vi "Kolmogan main.vi"(8 "Error In":errorcluster, 11 "Name":string) -> (0 "Error Out":errorcluster)   [LabVIEW 2019, in "Kolmogan Library 1.lvlib"]
uses:
  Kolmogan Library 1.lvlib
  <vilib>/NI/Modbus Library/API/Wrapper/Create TCP Master.vi
  <vilib>/regexp/Match Regular Expression.xnode
  <vilib>/NI/Modbus Library/API/Master/Modbus Master.lvclass
  Queue/Queue.lvlib
  Data Error Notifier/Data and Error Notifier.lvlib
  <vilib>/NI/Modbus Library/API/Wrapper/API Main.lvlib
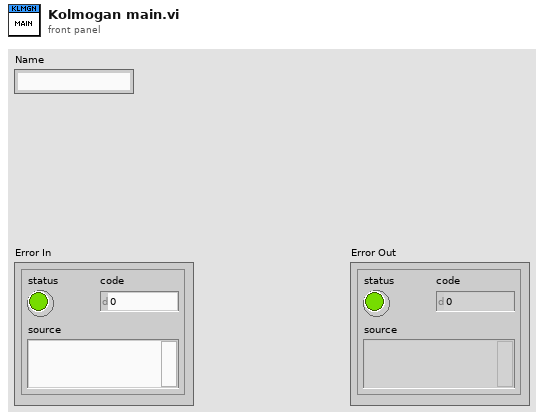
[diagram p1: front panel]
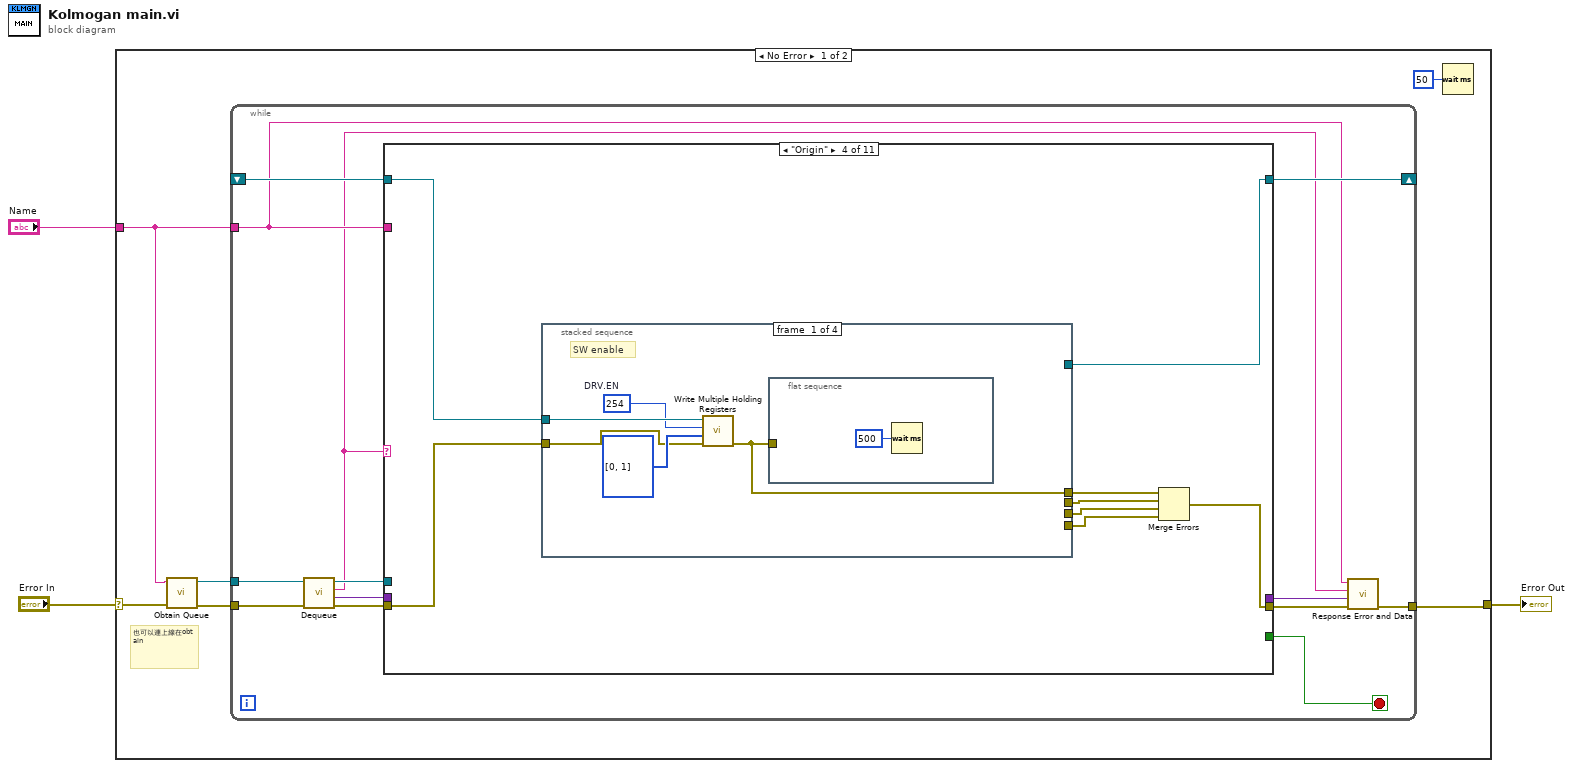
[diagram p0: block diagram]
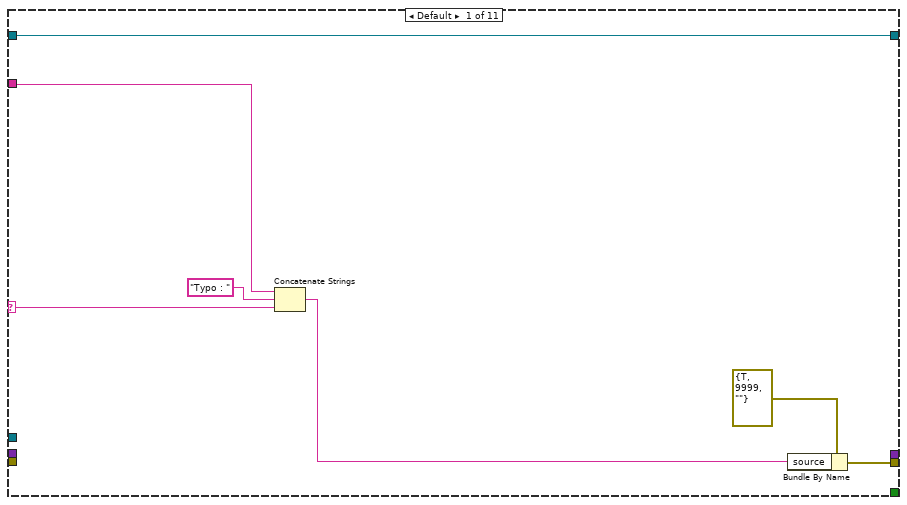
[diagram p2: hidden frame]
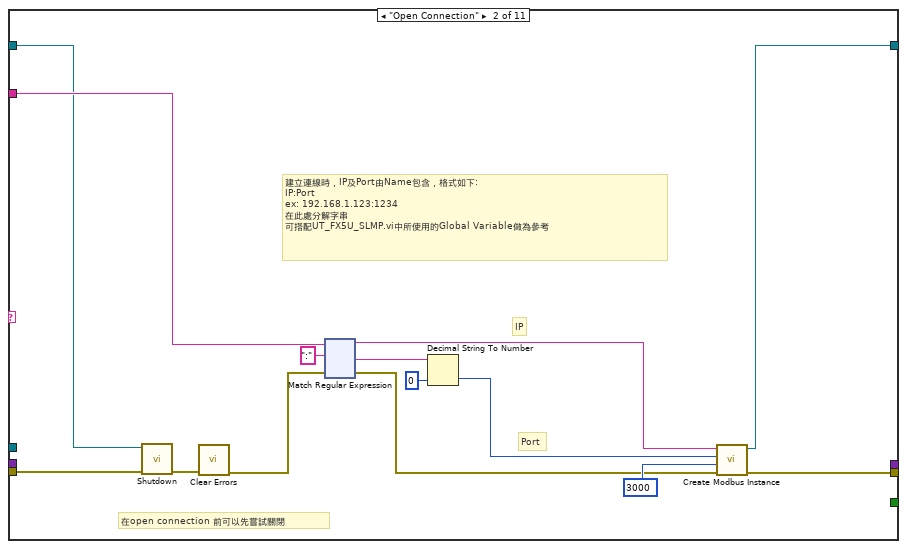
[diagram p3: hidden frame]
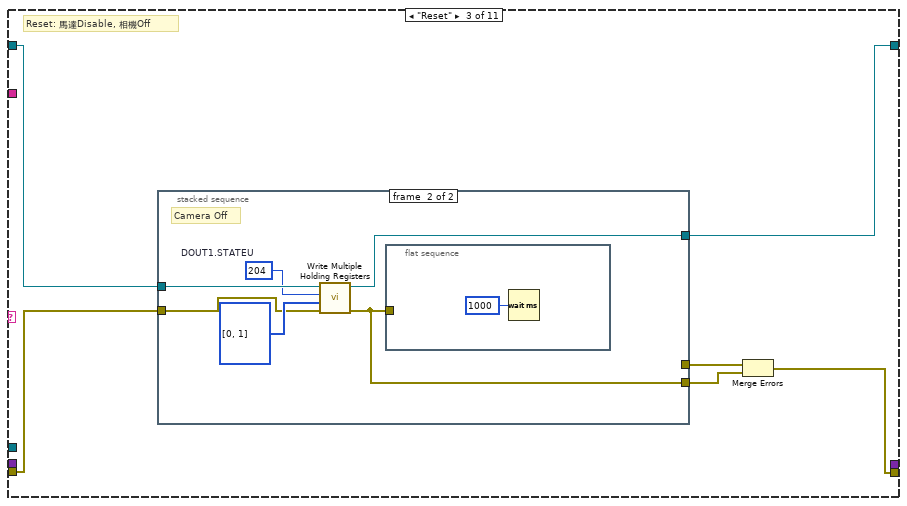
[diagram p4: hidden frame]
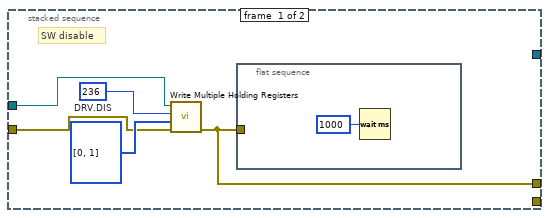
[diagram p5: hidden frame]
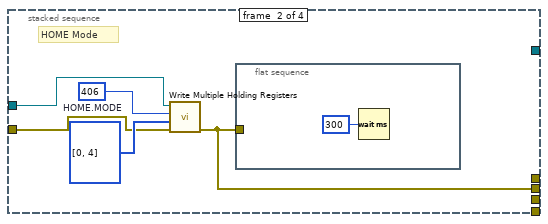
[diagram p6: hidden frame]
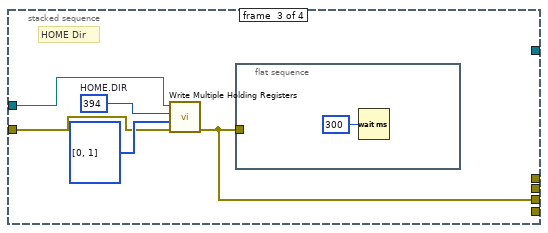
[diagram p7: hidden frame]
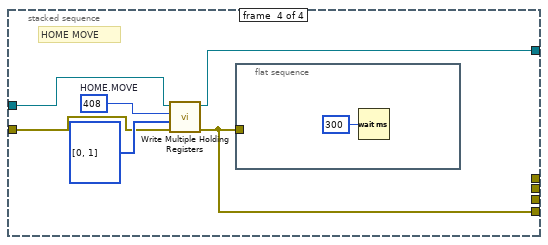
[diagram p8: hidden frame]
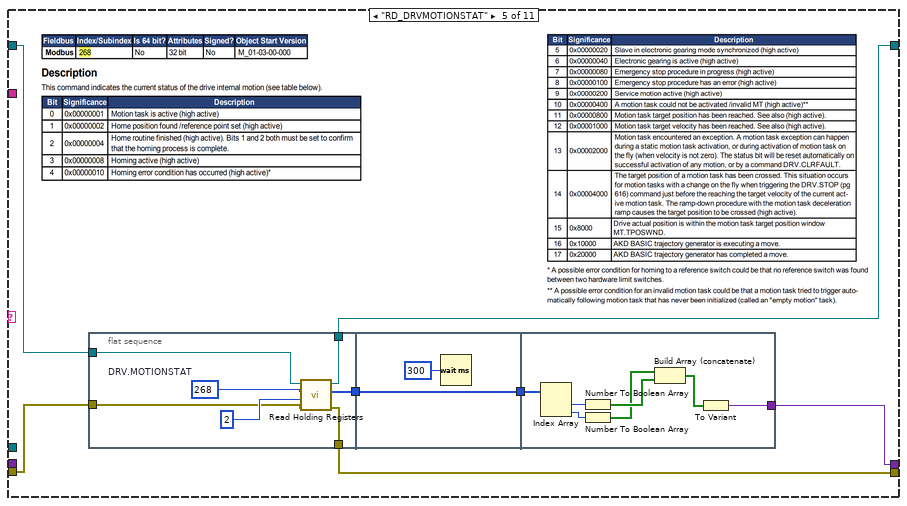
[diagram p9: hidden frame]
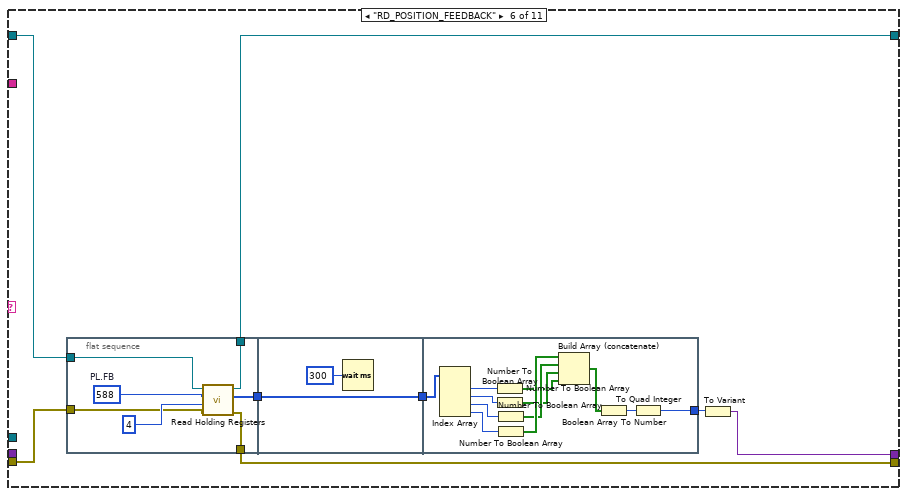
[diagram p10: hidden frame]
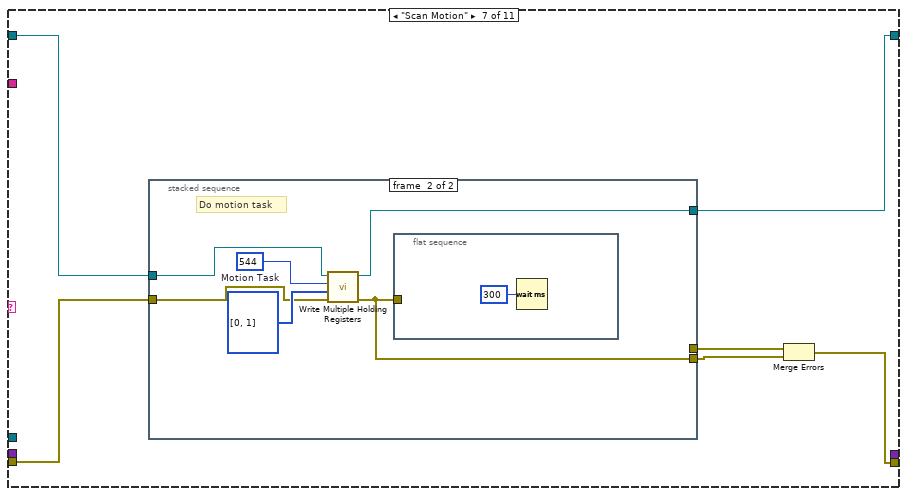
[diagram p11: hidden frame]
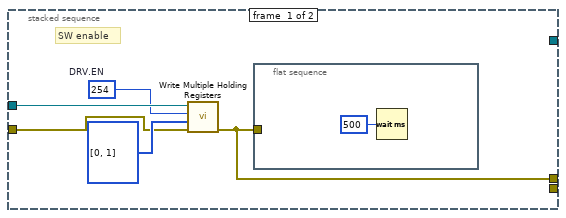
[diagram p12: hidden frame]
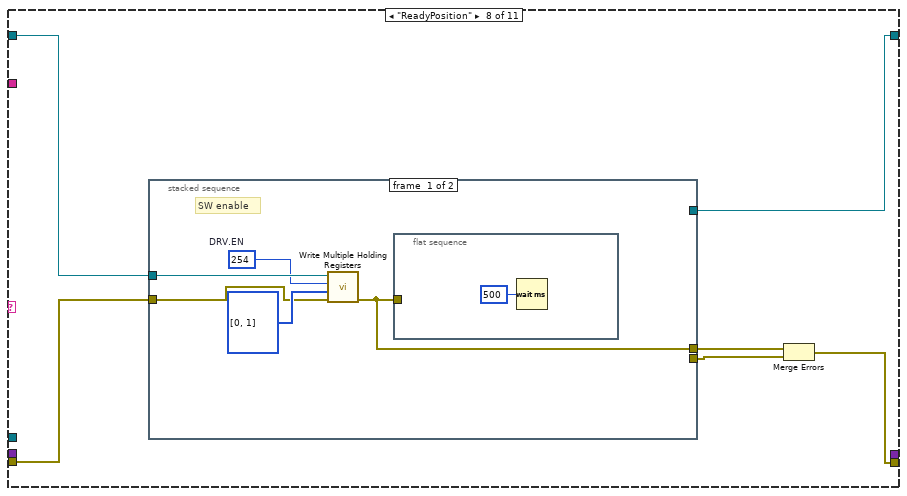
[diagram p13: hidden frame]
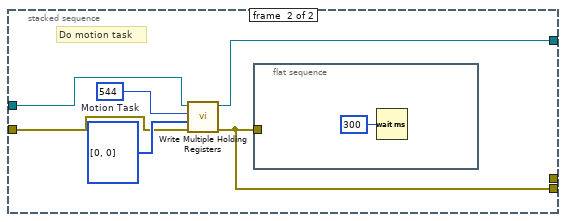
[diagram p14: hidden frame]
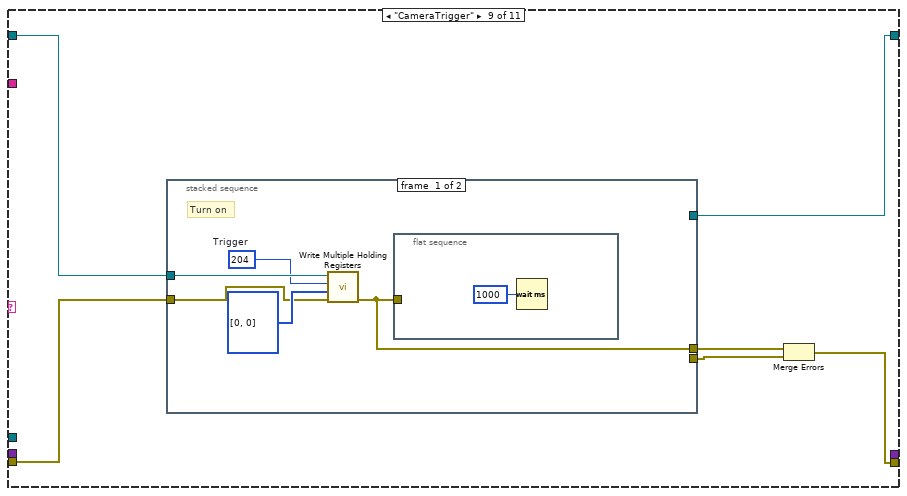
[diagram p15: hidden frame]
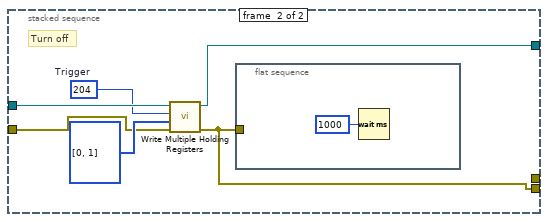
[diagram p16: hidden frame]
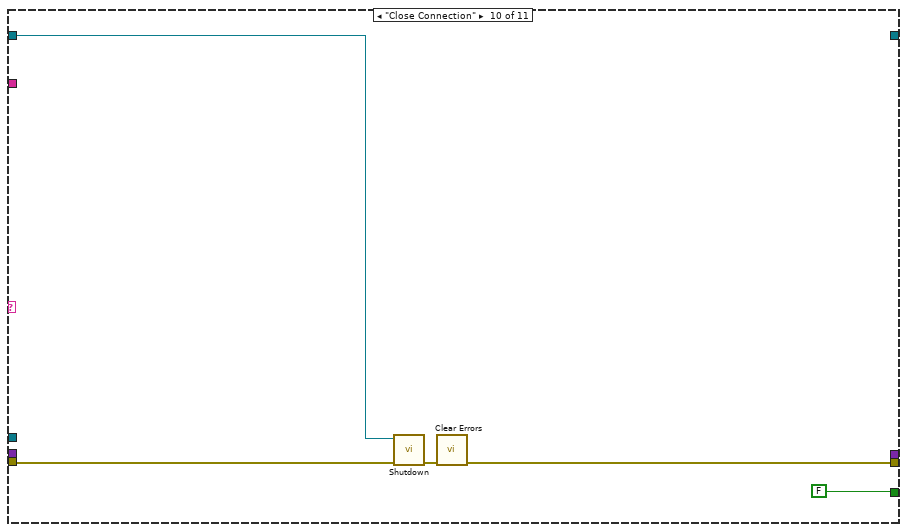
[diagram p17: hidden frame]
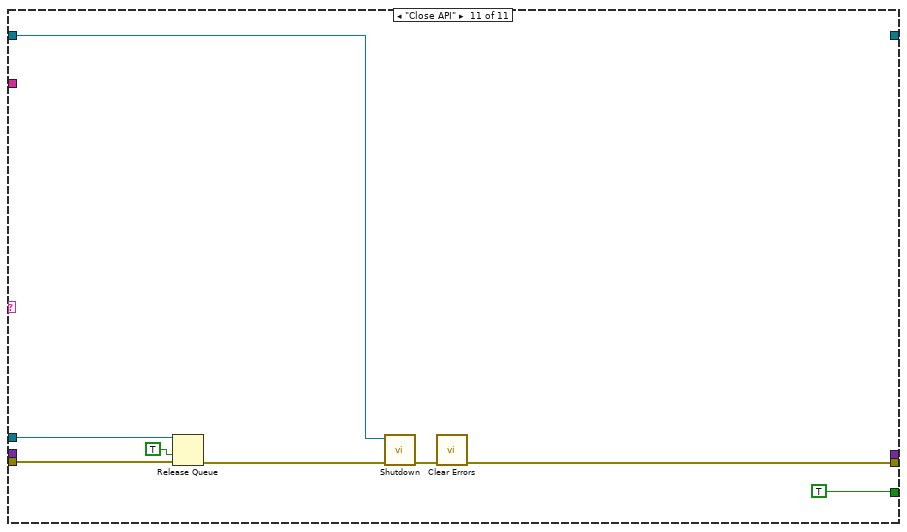
[diagram p18: hidden frame]
diagram:
  n1 = case shown="No Error" "Error In" {
    selector: "Error In" -> [w8 w332]
    tunnel: [w5 w332] -> w2
    tunnel: "Name" -> [w9 _]
    frame No Error {
      # "也可以連上線在obtain"
      n2 = call "Obtain Queue.vi"("Error In"=w8, "Name"=w9) -> ("Error Out"=w6:errorcluster, "queue out"=w7:refnum<queue>)  [unwired: 8 in]
      n3 = while {
        tunnel: w9 -> [w12]
        shift-right: [w22] -> _
        shift-left: _ -> [w21]
        tunnel: w7 -> [w19]
        tunnel: w6 -> [w18]
        tunnel: [w13] -> w5
        stop <- w20 stop-if-true
        n4 = call "Dequeue.vi"("Error In"=w18, "queue in"=w19) -> ("Error Out"=w16:errorcluster, "Data"=w15:variant, "Message"=w11:string, "queue out"=w17:refnum<queue>)  [unwired: 6 in]
        n5 = case shown="\"Origin\"" w11 {
          selector: w11 -> [w27 _ _ _ _ _ _ _ _ _ _]
          tunnel: w12 -> [w29 w40 _ _ _ _ _ _ _ _ _]
          tunnel: [w23 w34 w158 w177 w211 w236 w263 w282 w301 w322 w330] -> w14
          tunnel: [w26 w33 w161 w182 w210 w233 w262 w281 w300 _ _] -> w22
          tunnel: w21 -> [w26 w31 w163 w184 w216 w238 w267 w286 w305 w321 w326]
          tunnel: [_ _ _ _ _ _ _ _ _ FALSE TRUE] -> w20
          tunnel: w17 -> [_ _ _ _ _ _ _ _ _ _ w328]
          tunnel: w16 -> [_ w30 w162 w183 w215 w237 w266 w285 w304 w320 w327]
          tunnel: w15 -> [_ _ _ _ _ _ _ _ _ _ _]
          tunnel: [_ _ _ _ w214 w234 _ _ _ _ _] -> w10
          frame Default {
            n6 = Concatenate Strings(w29, "Typo : " ("string"), w27) -> (w24:string)
            n7 = Bundle By Name(cluster=errorcluster {"status"=TRUE, "code"=9999, "source"=""} ("error out"), "source"=w24) -> (w23:errorcluster)
          }
          frame "Open Connection" {
            # "建立連線時，IP及Port由Name包含，格式如下:\nIP:Port\nex: 192.168.1.123:1234\n在此處分解字串\n可搭配UT_FX5U_SLMP.vi中所使用的Global Variable做為參考"
            # "Port"
            # "IP"
            # "在open connection 前可以先嘗試關閉"
            n8 = call-dynamic "Shutdown.vi"("error in"=w30, "Modbus master in"=w31) -> ("error out"=w32:errorcluster)  [unwired: 9 in]
            n9 = call <vilib>:"Clear Errors.vi"("error in (no error)"=w32) -> ("error out"=w39:errorcluster)  [unwired: 5 in, 1 out]
            n10 = xnode "Match Regular Expression"("input string"=w40, "regular expression"=":", "error in"=w39) -> ("before match"=w38:string, "after match"=w42:string, "error out"=w35:errorcluster)  [unwired: 3 in, 2 out]
            n11 = Decimal String To Number(string=w42, default (0L)=u16 0 ("default (0 I32)")) -> (number=w37:u16)  [unwired: 1 in, 1 out]
            n12 = call-poly <vilib>:"Create Modbus Instance.vi"("error in"=w35, "connect timeout ms"=3000 ("timeout ms (60000)"), "port (502)"=w37, "address"=w38) -> ("error out"=w34:errorcluster, "TCP master instance"=w33:refnum<class "Modbus Master.lvclass">)  [unwired: 6 in]
          }
          frame "Reset" {
            # "Reset: 馬達Disable, 相機Off"
            n13 = stacked-sequence {
              tunnel: w163 -> [w168 w175]
              tunnel: w162 -> [w165 w172]
              tunnel: [_ w171] -> w161
              tunnel: [w164 _] -> w160
              tunnel: [_ w170] -> w159
              frame #0 {
                w167 = u16 236  # DRV.DIS
                # "SW disable"
                n14 = call-dynamic "Write Multiple Holding Registers.vi"("error in"=w165, "registers to write"=u16[] [0, 1], "starting address"=w167, "Modbus master in"=w168) -> ("error out"=w164:errorcluster)  [unwired: 6 in, 1 out]
                n15 = flat-sequence {
                  tunnel: w164 -> [_]
                  frame #0 {
                    n16 = Wait (ms)(milliseconds to wait=u32 1000) -> ()  [unwired: 1 out]
                  }
                }
              }
              frame #1 {
                w174 = u16 204  # DOUT1.STATEU
                # "Camera Off"
                n17 = call-dynamic "Write Multiple Holding Registers.vi"("error in"=w172, "registers to write"=u16[] [0, 1], "starting address"=w174, "Modbus master in"=w175) -> ("error out"=w170:errorcluster, "Modbus master out"=w171:refnum<class "Modbus Master.lvclass">)  [unwired: 6 in]
                n18 = flat-sequence {
                  tunnel: w170 -> [_]
                  frame #0 {
                    n19 = Wait (ms)(milliseconds to wait=u32 1000) -> ()  [unwired: 1 out]
                  }
                }
              }
            }
            n20 = Merge Errors(w160, w159) -> (w158:errorcluster)
          }
          frame "Origin" {
            n21 = stacked-sequence {
              tunnel: w184 -> [w189 w195 w201 w208]
              tunnel: w183 -> [w186 w192 w198 w205]
              tunnel: [_ _ _ w204] -> w182
              tunnel: [w185 _ _ _] -> w181
              tunnel: [_ w191 _ _] -> w180
              tunnel: [_ _ w197 _] -> w179
              tunnel: [_ _ _ w203] -> w178
              frame #0 {
                w188 = u16 254  # DRV.EN
                # "SW enable"
                n22 = call-dynamic "Write Multiple Holding Registers.vi"("error in"=w186, "registers to write"=u16[] [0, 1], "starting address"=w188, "Modbus master in"=w189) -> ("error out"=w185:errorcluster)  [unwired: 6 in, 1 out]
                n23 = flat-sequence {
                  tunnel: w185 -> [_]
                  frame #0 {
                    n24 = Wait (ms)(milliseconds to wait=u32 500) -> ()  [unwired: 1 out]
                  }
                }
              }
              frame #1 {
                w194 = u16 406  # HOME.MODE
                # "HOME Mode"
                n25 = call-dynamic "Write Multiple Holding Registers.vi"("error in"=w192, "registers to write"=u16[] [0, 4], "starting address"=w194, "Modbus master in"=w195) -> ("error out"=w191:errorcluster)  [unwired: 6 in, 1 out]
                n26 = flat-sequence {
                  tunnel: w191 -> [_]
                  frame #0 {
                    n27 = Wait (ms)(milliseconds to wait=u32 300) -> ()  [unwired: 1 out]
                  }
                }
              }
              frame #2 {
                w200 = u16 394  # HOME.DIR
                # "HOME Dir"
                n28 = call-dynamic "Write Multiple Holding Registers.vi"("error in"=w198, "registers to write"=u16[] [0, 1], "starting address"=w200, "Modbus master in"=w201) -> ("error out"=w197:errorcluster)  [unwired: 6 in, 1 out]
                n29 = flat-sequence {
                  tunnel: w197 -> [_]
                  frame #0 {
                    n30 = Wait (ms)(milliseconds to wait=u32 300) -> ()  [unwired: 1 out]
                  }
                }
              }
              frame #3 {
                w207 = u16 408  # HOME.MOVE
                # "HOME MOVE"
                n31 = call-dynamic "Write Multiple Holding Registers.vi"("error in"=w205, "registers to write"=u16[] [0, 1], "starting address"=w207, "Modbus master in"=w208) -> ("error out"=w203:errorcluster, "Modbus master out"=w204:refnum<class "Modbus Master.lvclass">)  [unwired: 6 in]
                n32 = flat-sequence {
                  tunnel: w203 -> [_]
                  frame #0 {
                    n33 = Wait (ms)(milliseconds to wait=u32 300) -> ()  [unwired: 1 out]
                  }
                }
              }
            }
            n34 = Merge Errors(w181, w180, w179, w178) -> (w177:errorcluster)
          }
          frame "RD_DRVMOTIONSTAT" {
            n35 = flat-sequence {
              tunnel: w216 -> [w220]
              tunnel: w215 -> [w219]
              tunnel: [w221] -> w213
              tunnel: [w218] -> w211
              tunnel: [w217] -> w210
              tunnel: w213 -> [w225]
              tunnel: [w225] -> w212
              tunnel: w212 -> [w227]
              tunnel: [w226] -> w214
              frame #0 {
                w223 = u16 268  # DRV.MOTIONSTAT
                n36 = call-dynamic "Read Holding Registers.vi"("error in"=w219, "number of inputs"=u16 2, "starting address"=w223, "Modbus master in"=w220) -> ("error out"=w218:errorcluster, "register values"=w221:u16[], "Modbus master out"=w217:refnum<class "Modbus Master.lvclass">)  [unwired: 5 in]
              }
              frame #1 {
                n37 = Wait (ms)(milliseconds to wait=u32 300) -> ()  [unwired: 1 out]
              }
              frame #2 {
                n38 = Index Array(array=w227) -> (element #1=w228:u16, element #2=w229:u16)  [unwired: 2 in]
                n39 = Number To Boolean Array(number=w228) -> (Boolean array=w231:bool[])
                n40 = Number To Boolean Array(number=w229) -> (Boolean array=w230:bool[])
                n41 = Build Array (concatenate)(w230, w231) -> (w232:bool[])
                n42 = To Variant(anything=w232) -> (Variant=w226:variant)
              }
            }
          }
          frame "RD_POSITION_FEEDBACK" {
            n43 = flat-sequence {
              tunnel: w238 -> [w244]
              tunnel: w237 -> [w243]
              tunnel: [w245] -> w240
              tunnel: [w242] -> w236
              tunnel: [w241] -> w233
              tunnel: w240 -> [w249]
              tunnel: [w249] -> w239
              tunnel: w239 -> [w259]
              tunnel: [w250] -> w235
              frame #0 {
                w247 = u16 588  # PL.FB
                n44 = call-dynamic "Read Holding Registers.vi"("error in"=w243, "number of inputs"=u16 4, "starting address"=w247, "Modbus master in"=w244) -> ("error out"=w242:errorcluster, "register values"=w245:u16[], "Modbus master out"=w241:refnum<class "Modbus Master.lvclass">)  [unwired: 5 in]
              }
              frame #1 {
                n45 = Wait (ms)(milliseconds to wait=u32 300) -> ()  [unwired: 1 out]
              }
              frame #2 {
                n46 = Index Array(array=w259) -> (element #1=w260:u16, element #2=w261:u16, element #3=w258:u16, element #4=w257:u16)  [unwired: 4 in]
                n47 = Number To Boolean Array(number=w260) -> (Boolean array=w253:bool[])
                n48 = Number To Boolean Array(number=w261) -> (Boolean array=w254:bool[])
                n49 = Number To Boolean Array(number=w258) -> (Boolean array=w255:bool[])
                n50 = Number To Boolean Array(number=w257) -> (Boolean array=w256:bool[])
                n51 = Build Array (concatenate)(w256, w255, w254, w253) -> (w252:bool[])
                n52 = Boolean Array To Number(Boolean array=w252) -> (number=w251:u32)
                n53 = To Quad Integer(1:w251) -> (0:w250:i64)
              }
            }
            n54 = To Variant(anything=w235) -> (Variant=w234:variant)
          }
          frame "Scan Motion" {
            n55 = stacked-sequence {
              tunnel: w267 -> [w272 w279]
              tunnel: w266 -> [w269 w276]
              tunnel: [w268 _] -> w265
              tunnel: [_ w275] -> w264
              tunnel: [_ w274] -> w262
              frame #0 {
                w271 = u16 254  # DRV.EN
                # "SW enable"
                n56 = call-dynamic "Write Multiple Holding Registers.vi"("error in"=w269, "registers to write"=u16[] [0, 1], "starting address"=w271, "Modbus master in"=w272) -> ("error out"=w268:errorcluster)  [unwired: 6 in, 1 out]
                n57 = flat-sequence {
                  tunnel: w268 -> [_]
                  frame #0 {
                    n58 = Wait (ms)(milliseconds to wait=u32 500) -> ()  [unwired: 1 out]
                  }
                }
              }
              frame #1 {
                w278 = u16 544  # Motion Task
                # "Do motion task"
                n59 = call-dynamic "Write Multiple Holding Registers.vi"("error in"=w276, "registers to write"=u16[] [0, 1], "starting address"=w278, "Modbus master in"=w279) -> ("error out"=w275:errorcluster, "Modbus master out"=w274:refnum<class "Modbus Master.lvclass">)  [unwired: 6 in]
                n60 = flat-sequence {
                  tunnel: w275 -> [_]
                  frame #0 {
                    n61 = Wait (ms)(milliseconds to wait=u32 300) -> ()  [unwired: 1 out]
                  }
                }
              }
            }
            n62 = Merge Errors(w265, w264) -> (w263:errorcluster)
          }
          frame "ReadyPosition" {
            n63 = stacked-sequence {
              tunnel: w286 -> [w291 w298]
              tunnel: w285 -> [w288 w295]
              tunnel: [w287 _] -> w284
              tunnel: [_ w294] -> w283
              tunnel: [_ w293] -> w281
              frame #0 {
                w290 = u16 254  # DRV.EN
                # "SW enable"
                n64 = call-dynamic "Write Multiple Holding Registers.vi"("error in"=w288, "registers to write"=u16[] [0, 1], "starting address"=w290, "Modbus master in"=w291) -> ("error out"=w287:errorcluster)  [unwired: 6 in, 1 out]
                n65 = flat-sequence {
                  tunnel: w287 -> [_]
                  frame #0 {
                    n66 = Wait (ms)(milliseconds to wait=u32 500) -> ()  [unwired: 1 out]
                  }
                }
              }
              frame #1 {
                w297 = u16 544  # Motion Task
                # "Do motion task"
                n67 = call-dynamic "Write Multiple Holding Registers.vi"("error in"=w295, "registers to write"=u16[] [0, 0], "starting address"=w297, "Modbus master in"=w298) -> ("error out"=w294:errorcluster, "Modbus master out"=w293:refnum<class "Modbus Master.lvclass">)  [unwired: 6 in]
                n68 = flat-sequence {
                  tunnel: w294 -> [_]
                  frame #0 {
                    n69 = Wait (ms)(milliseconds to wait=u32 300) -> ()  [unwired: 1 out]
                  }
                }
              }
            }
            n70 = Merge Errors(w284, w283) -> (w282:errorcluster)
          }
          frame "CameraTrigger" {
            n71 = stacked-sequence {
              tunnel: w305 -> [w310 w317]
              tunnel: w304 -> [w307 w314]
              tunnel: [w306 _] -> w303
              tunnel: [_ w313] -> w302
              tunnel: [_ w312] -> w300
              frame #0 {
                w309 = u16 204  # Trigger
                # "Turn on"
                n72 = call-dynamic "Write Multiple Holding Registers.vi"("error in"=w307, "registers to write"=u16[] [0, 0], "starting address"=w309, "Modbus master in"=w310) -> ("error out"=w306:errorcluster)  [unwired: 6 in, 1 out]
                n73 = flat-sequence {
                  tunnel: w306 -> [_]
                  frame #0 {
                    n74 = Wait (ms)(milliseconds to wait=u32 1000) -> ()  [unwired: 1 out]
                  }
                }
              }
              frame #1 {
                w316 = u16 204  # Trigger
                # "Turn off"
                n75 = call-dynamic "Write Multiple Holding Registers.vi"("error in"=w314, "registers to write"=u16[] [0, 1], "starting address"=w316, "Modbus master in"=w317) -> ("error out"=w313:errorcluster, "Modbus master out"=w312:refnum<class "Modbus Master.lvclass">)  [unwired: 6 in]
                n76 = flat-sequence {
                  tunnel: w313 -> [_]
                  frame #0 {
                    n77 = Wait (ms)(milliseconds to wait=u32 1000) -> ()  [unwired: 1 out]
                  }
                }
              }
            }
            n78 = Merge Errors(w303, w302) -> (w301:errorcluster)
          }
          frame "Close Connection" {
            n79 = call-dynamic "Shutdown.vi"("error in"=w320, "Modbus master in"=w321) -> ("error out"=w319:errorcluster)  [unwired: 9 in]
            n80 = call <vilib>:"Clear Errors.vi"("error in (no error)"=w319) -> ("error out"=w322:errorcluster)  [unwired: 5 in, 1 out]
          }
          frame "Close API" {
            n81 = Release Queue(queue=w328, force destroy? (F)=TRUE, error in (no error)=w327) -> (error out=w325:errorcluster)  [unwired: 2 out]
            n82 = call-dynamic "Shutdown.vi"("error in"=w325, "Modbus master in"=w326) -> ("error out"=w324:errorcluster)  [unwired: 9 in]
            n83 = call <vilib>:"Clear Errors.vi"("error in (no error)"=w324) -> ("error out"=w330:errorcluster)  [unwired: 5 in, 1 out]
          }
        }
        n84 = call "Response Error and Data.vi"("error in (no error)"=w14, "Data In"=w10, "Message"=w11, "Name"=w12) -> ("error out"=w13:errorcluster)  [unwired: 5 in, 2 out]
      }
      n85 = Wait (ms)(milliseconds to wait=u32 50) -> ()  [unwired: 1 out]
    }
    frame Error {
    }
  }
  "Error Out" <- w2
